vi "Pointer producer consumer Motor Code n Graph.vi"(7 "error in (no error)":errorcluster, 10 "DecimalMotorCode":i32) -> (0 "error IO":errorcluster, 1 "Motor":cluster{dbl, i16}(graph), 2 "Motor Array":bool[](array[boolean]), 3 "MotorSubarray":i16[](array[numeric]))   [LabVIEW 2014]
panel:
  # "Code 1 = X -1\nCode 2 = X +1\nCode 4 = O +1\nCode 8 = O -1"
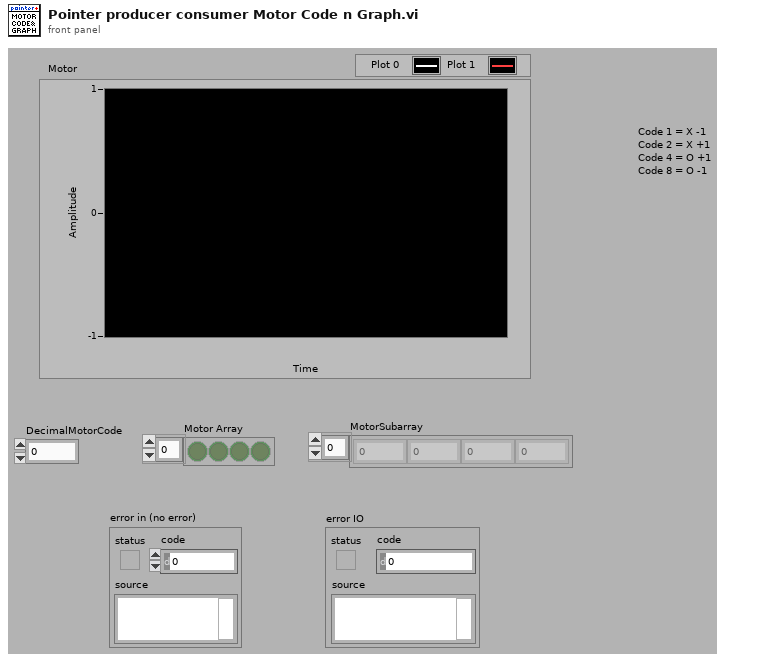
[diagram p1: front panel]
types:
  T1 = cluster{"[0]":i16, "[1]":i16, "[2]":i16, "[3]":i16, "[4]":i16, "[5]":i16, "[6]":i16, "[7]":i16, "[8]":i16}
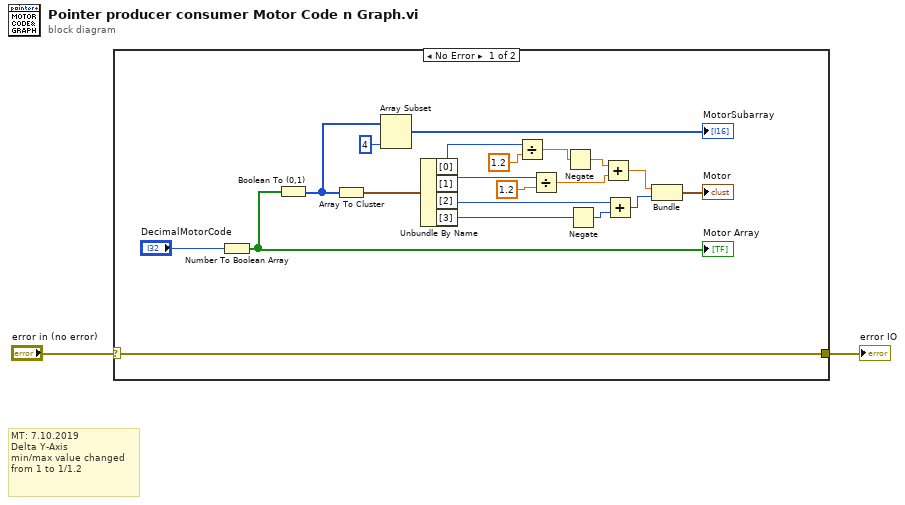
[diagram p0: block diagram]
diagram:
  # "MT: 7.10.2019\nDelta Y-Axis \nmin/max value changed from 1 to 1/1.2"
  n1 = case shown="No Error" "error in (no error)" {
    selector: "error in (no error)" -> [w9 w23]
    tunnel: [w9 w23] -> w1
    frame No Error {
      n2 = Number To Boolean Array(number="DecimalMotorCode") -> (Boolean array=w11:bool[])
      "Motor Array" <- w11
      n3 = Boolean To (0,1)(Boolean=w11) -> (0, 1=w20:i16[])
      n4 = Array To Cluster(array=w20) -> (cluster=w12:T1)
      n5 = Array Subset(array=w20, length=4) -> (→"MotorSubarray":i16[])  [unwired: 1 in]
      n6 = Unbundle By Name(w12) -> ("[0]"=w8:i16, "[1]"=w7:i16, "[2]"=w16:i16, "[3]"=w13:i16)
      n7 = Divide(x=w8, y=1.2) -> (x/y=w3:dbl)
      n8 = Divide(x=w7, y=1.2) -> (x/y=w4:dbl)
      n9 = Negate(x=w3) -> (-x=w14:dbl)
      n10 = Negate(x=w13) -> (-x=w15:i16)
      n11 = Add(x=w14, y=w4) -> (x+y=w18:dbl)
      n12 = Add(x=w16, y=w15) -> (x+y=w17:i16)
      n13 = Bundle(w18, w17) -> (→"Motor":cluster{dbl, i16})  [unwired: 1 in]
    }
    frame Error {
    }
  }
  "error IO" <- w1
